vi "Rising Edge.vi"(11 "signal":bool) -> (3 "rising edge":bool)   [LabVIEW 2017]
doc: "Returns TRUE for one call when signal changes from FALSE to TRUE."
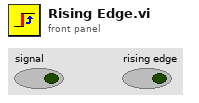
[diagram p1: front panel]
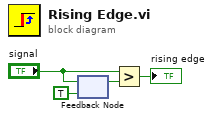
[diagram p0: block diagram]
diagram:
  n1 = feedback #1(TRUE ("signal")) -> (w2:bool)
  n2 = feedback-in #1("signal") -> ()
  n3 = Greater?(x="signal", y=w2) -> (0:→"rising edge":bool)
